vi "Activate Joystick.vi"(8 "error in (no error)":errorcluster, 11 "Gantry Class in":refnum<class "Gantry.lvclass">) -> (0 "error out":errorcluster, 3 "Gantry Class out":refnum<class "Gantry.lvclass">)   [LabVIEW 2026, in "Gantry.lvclass"]
uses:
  Gantry.lvclass
  <instrlib>/Aerotech Automation1/Aerotech Automation1.lvlib
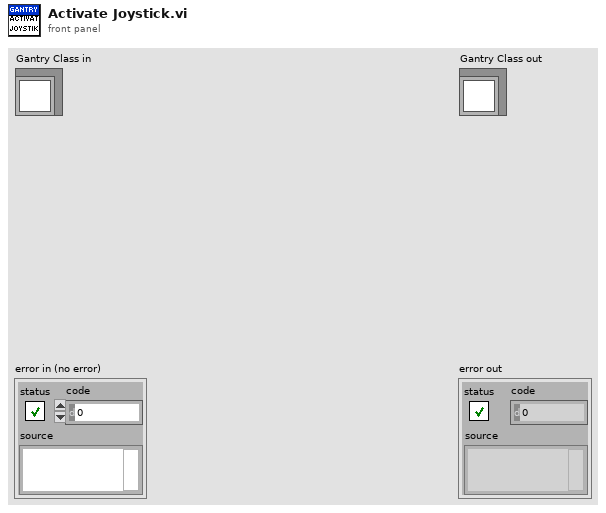
[diagram p1: front panel]
types:
  T1 = typedef "Virtual Modes.ctl" = enum16{"Nonvirtual", "Virtual"}
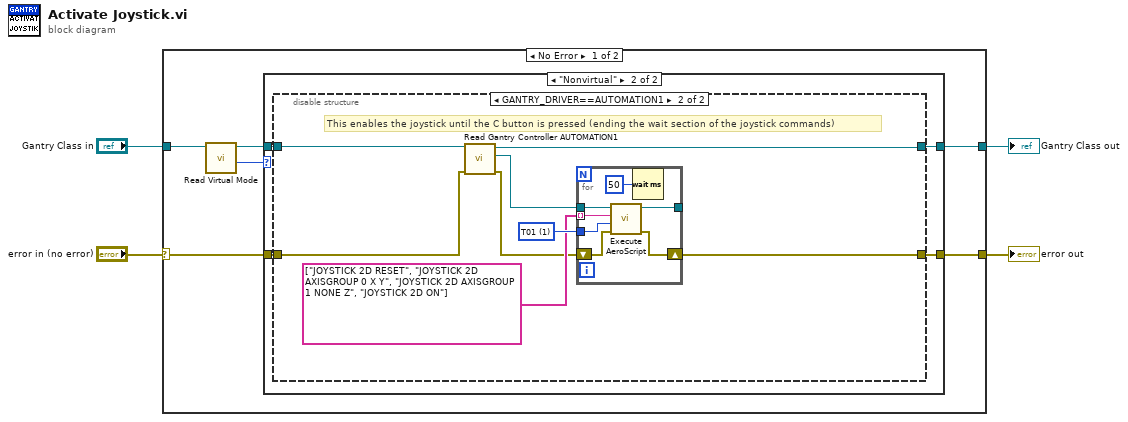
[diagram p0: block diagram]
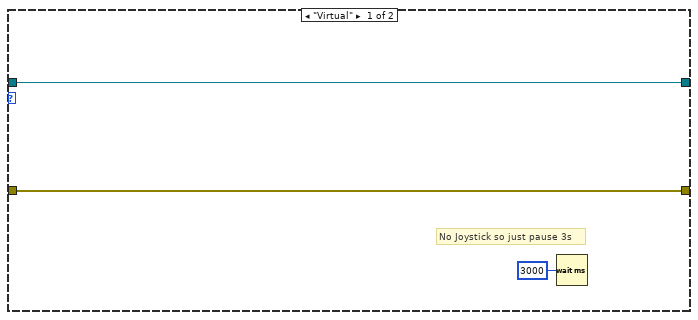
[diagram p2: hidden frame]
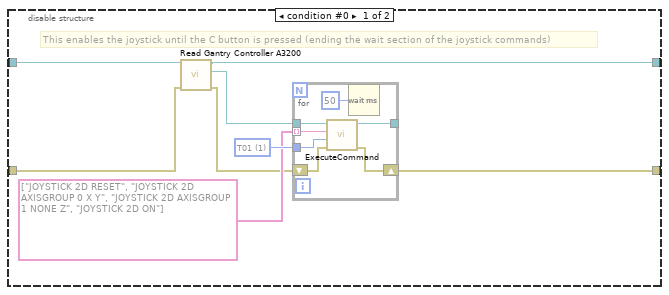
[diagram p3: hidden frame]
diagram:
  n1 = case shown="No Error" "error in (no error)" {
    selector: "error in (no error)" -> [w10 w49]
    tunnel: [w9 w49] -> w3
    tunnel: [w8 w48] -> w1
    tunnel: "Gantry Class in" -> [w7 w48]
    frame No Error {
      n2 = call-dynamic "Read Virtual Mode.vi"("Gantry in"=w7) -> ("Virtual Mode"=w5:T1, "Gantry out"=w6:refnum<class "Gantry.lvclass">)  [unwired: 7 in, 2 out]
      n3 = case shown="\"Nonvirtual\"" w5 {
        tunnel: w10 -> [w12 w15]
        tunnel: [w12 w17] -> w9
        tunnel: w6 -> [w13 w16]
        tunnel: [w13 w14] -> w8
        frame "Virtual" {
          # "No Joystick so just pause 3s"
          n4 = Wait (ms)(milliseconds to wait=u32 3000) -> ()  [unwired: 1 out]
        }
        frame "Nonvirtual" {
          n5 = disable-structure shown="GANTRY_DRIVER==AUTOMATION1" {
            disable-tunnel: [w23 w34] -> w17
            disable-tunnel: w16 -> [w22 w36]
            disable-tunnel: w15 -> [w21 w35]
            disable-tunnel: [w18 w33] -> w14
            frame condition #0 {
              w25 = 1 items=["TLibrary", "T01", "T02", "T03", "T04", "T05", "T06", "T07", "T08", "T09", "T10", "T11", "T12", "T13", "T14", "T15", "T16", "T17", "T18", "T19", "T20", "T21", "T22", "T23", "T24", "T25", "T26", "T27", "T28", "T29", "T30", "T31"] ("taskId")
              # "This enables the joystick until the C button is pressed (ending the wait section of the joystick commands)"
              n6 = call "Read Gantry Controller A3200.vi"("error in (no error)"=w21, "Gantry in"=w22) -> ("error out"=w20:errorcluster, "A3200 controller out"=w19:refnum<k24>, "Gantry out"=w18:refnum<class "Gantry.lvclass">)  [unwired: 7 in]
              n7 = for {
                shift-right: [w31] -> w23
                shift-left: w20 -> [w32]
                tunnel: w25 -> [w28]
                tunnel: w19 -> [w30]
                tunnel: [w29] -> _
                tunnel: string[] ["JOYSTICK 2D RESET", "JOYSTICK 2D AXISGROUP 0 X Y", "JOYSTICK 2D AXISGROUP 1 NONE Z", "JOYSTICK 2D ON"] -> [w27] mode=indexing
                n8 = call "ExecuteCommand.vi"("error in (no error)"=w32, "taskId"=w28, "Command Code"=w27, "controller in"=w30) -> ("error out"=w31:errorcluster, "controller out"=w29:refnum<k24>)  [unwired: 5 in, 1 out]
                n9 = Wait (ms)(milliseconds to wait=u32 50) -> ()  [unwired: 1 out]
              }
            }
            frame condition #1 (active) {
              w40 = 1 items=["TLibrary", "T01", "T02", "T03", "T04", "T05", "T06", "T07", "T08", "T09", "T10", "T11", "T12", "T13", "T14", "T15", "T16", "T17", "T18", "T19", "T20", "T21", "T22", "T23", "T24", "T25", "T26", "T27", "T28", "T29", "T30", "T31"] ("taskId")
              # "This enables the joystick until the C button is pressed (ending the wait section of the joystick commands)"
              n10 = call "Read Gantry Controller AUTOMATION1.vi"("error in (no error)"=w35, "Gantry in"=w36) -> ("error out"=w38:errorcluster, "Controller AUTOMATION1"=w37:refnum<k24>, "Gantry out"=w33:refnum<class "Gantry.lvclass">)  [unwired: 7 in]
              n11 = for {
                shift-right: [w46] -> w34
                shift-left: w38 -> [w47]
                tunnel: w40 -> [w43]
                tunnel: w37 -> [w45]
                tunnel: [w44] -> _
                tunnel: string[] ["JOYSTICK 2D RESET", "JOYSTICK 2D AXISGROUP 0 X Y", "JOYSTICK 2D AXISGROUP 1 NONE Z", "JOYSTICK 2D ON"] -> [w42] mode=indexing
                n12 = call <instrlib>:"Execute AeroScript.vi"("error in (no error)"=w47, "Task Index"=w43, "AeroScript Command"=w42, "Controller Refnum"=w45) -> ("error out"=w46:errorcluster, "Controller Refnum out"=w44:refnum<k24>)  [unwired: 6 in]
                n13 = Wait (ms)(milliseconds to wait=u32 50) -> ()  [unwired: 1 out]
              }
            }
          }
        }
      }
    }
    frame Error {
    }
  }
  "error out" <- w3
  "Gantry Class out" <- w1
